vi "Configure Amplitude Characteristics.vi"(0 "VISA resource name":refnum<visa-resource-name>, 1 "Internal Preamp (0: Off)":i32(ring) items=["Off", "Low Band", "Full Range"], 5 "Enable Presel Center (T: Enable)":bool=TRUE, 7 "Presel Adjust (0 Hz)":dbl, 9 "Max Mixer Level  (-10 dBm)":dbl=-10.0, 11 "error in (no error)":errorcluster, 12 "uw Path Control (0: Off)":i32(ring) items=["Standard Path", "Low Noise Path", "Preselector Bypass"]) -> (4 "VISA resource name out":refnum<visa-resource-name>, 15 "error out":errorcluster)   [LabVIEW 2018, in "Agilent MXA Series.lvlib"]
doc: "Configures Preselector, Internal Preamp and Max Mixer Level."
uses:
  Agilent MXA Series.lvlib
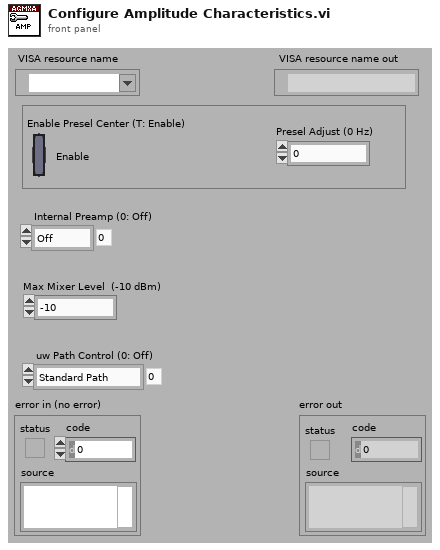
[diagram p1: front panel]
types:
  T1 = typedef "Agilent MXA Series.lvlib/Extended User Data.ctl" = cluster{"Measurement Type":i32, "Agilent MXA/EXA Model":i32}
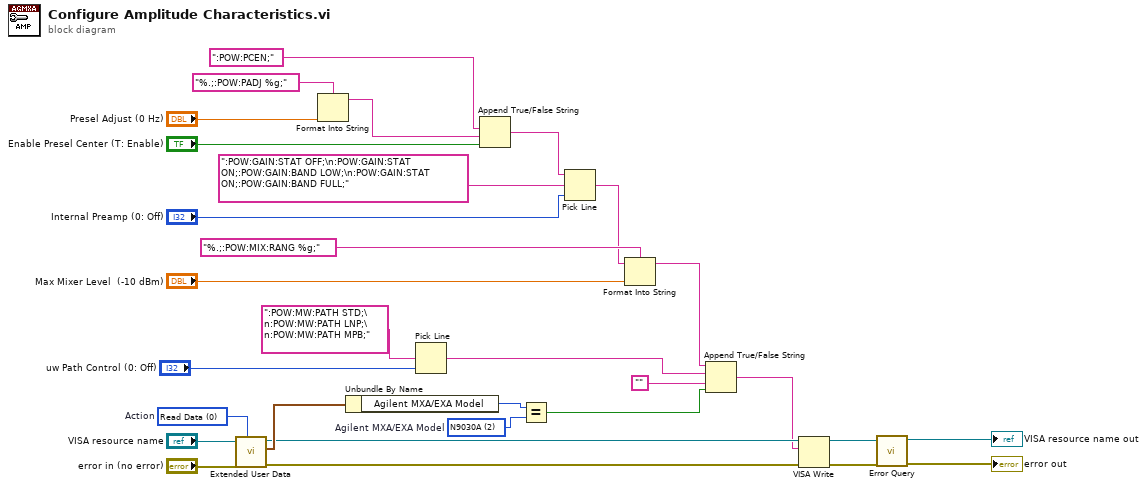
[diagram p0: block diagram]
diagram:
  w8 = 2 items=["N9020A", "N9010A", "N9030A", "N9000A"]  # Agilent MXA/EXA Model
  w11 = 0 items=["Read Data", "Write Data", "Clear Data", "Clear ALL Data"]  # Action
  n1 = call "Extended User Data.vi"("Action (1:Write Data)"=w11, "Error In (no error)"="error in (no error)", "VISA resource name in"="VISA resource name") -> ("Error Out"=w6:errorcluster, "User Data Out"=w10:T1, "VISA resource name out"=w7:refnum<visa-resource-name>)  [unwired: 6 in]
  n2 = Format Into String(format string="%.;:POW:PADJ %g;", "Presel Adjust (0 Hz)") -> (resulting string=w27:string)  [unwired: 2 in, 1 out]
  n3 = Unbundle By Name(w10) -> ("Agilent MXA/EXA Model"=w9:i32)
  n4 = Pick Line(multi-line string=":POW:MW:PATH STD;\n:POW:MW:PATH LNP;\n:POW:MW:PATH MPB;", line index="uw Path Control (0: Off)") -> (output string=w4:string)  [unwired: 1 in]
  n5 = Append True/False String(1:"Enable Presel Center (T: Enable)", 2:w27, 3:":POW:PCEN;" ("true string")) -> (0:w23:string)  [unwired: 1 in]
  n6 = Equal?(x=w9, y=w8) -> (x = y?=w5:bool)
  n7 = Pick Line(string ("")=w23, multi-line string=":POW:GAIN:STAT OFF;\n:POW:GAIN:STAT ON;:POW:GAIN:BAND LOW;\n:POW:GAIN:STAT ON;:POW:GAIN:BAND FULL;", line index="Internal Preamp (0: Off)") -> (output string=w20:string)
  n8 = Format Into String(format string="%.;:POW:MIX:RANG %g;", initial string=w20, "Max Mixer Level  (-10 dBm)") -> (resulting string=w3:string)  [unwired: 1 in, 1 out]
  n9 = Append True/False String(1:w5, 2:"", 3:w4, 4:w3) -> (0:w1:string)
  n10 = VISA Write(VISA resource name=w7, write buffer=w1, error in (no error)=w6) -> (VISA resource name out=w18:refnum<visa-resource-name>, error out=w19:errorcluster)  [unwired: 1 out]
  n11 = call "Error Query.vi"("error in (no error)"=w19, "VISA resource name"=w18) -> ("error out"=→"error out":errorcluster, "VISA resource name out"=→"VISA resource name out":refnum<visa-resource-name>)  [unwired: 6 in, 2 out]
